vi "Avantes - AVS_PrepareMeasure.vi"(8 "error in (no error)":errorcluster, 11 "Cluster in":T1) -> (0 "error out":errorcluster, 3 "Cluster out":T1)   [LabVIEW 2013, in "Avantes Spectrometer Functions.lvlib"]
uses:
  Avantes Spectrometer Functions.lvlib
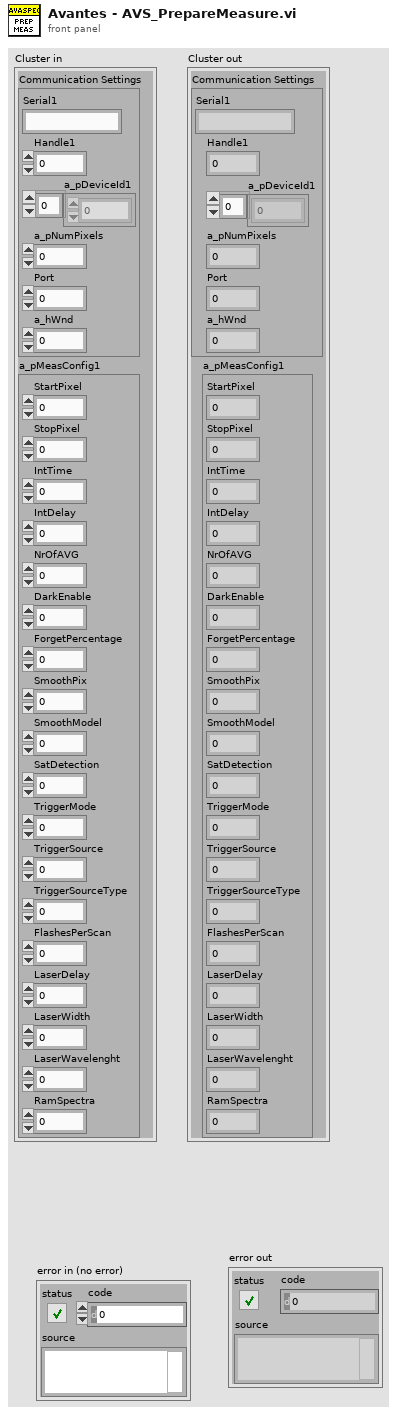
[diagram p1: front panel]
types:
  T1 = cluster{"Communication Settings":cluster{"Serial1":string, "Handle1":i32, "a_pDeviceId1":u8[], "a_pNumPixels":u16, "Port":i32, "a_hWnd":i32}, "a_pMeasConfig1":cluster{"StartPixel":u16, "StopPixel":u16, "IntTime":sgl, "IntDelay":u32, "NrOfAVG":u32, "DarkEnable":u8, "ForgetPercentage":u8, "SmoothPix":u16, "SmoothModel":u8, "SatDetection":u8, "TriggerMode":u8, "TriggerSource":u8, "TriggerSourceType":u8, "FlashesPerScan":u16, "LaserDelay":u32, "LaserWidth":u32, "LaserWavelenght":sgl, "RamSpectra":u16}}
  T2 = cluster{"StartPixel":u16, "StopPixel":u16, "IntTime":sgl, "IntDelay":u32, "NrOfAVG":u32, "DarkEnable":u8, "ForgetPercentage":u8, "SmoothPix":u16, "SmoothModel":u8, "SatDetection":u8, "TriggerMode":u8, "TriggerSource":u8, "TriggerSourceType":u8, "FlashesPerScan":u16, "LaserDelay":u32, "LaserWidth":u32, "LaserWavelenght":sgl, "RamSpectra":u16}
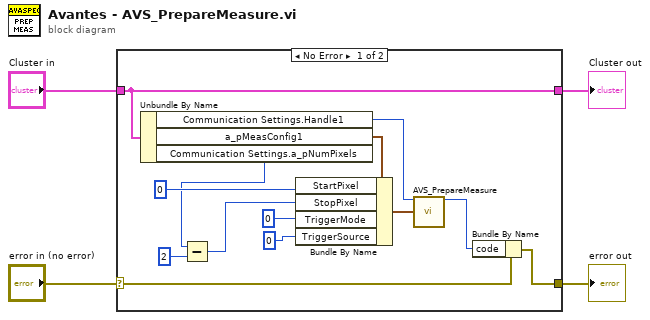
[diagram p0: block diagram]
diagram:
  n1 = case shown="No Error" "error in (no error)" {
    selector: "error in (no error)" -> [w10 w19]
    tunnel: [w11 w18] -> w4
    tunnel: "Cluster in" -> [w11 w18]
    tunnel: [w9 w19] -> w1
    frame No Error {
      n2 = Unbundle By Name(w11) -> ("Communication Settings.Handle1"=w6:i32, "a_pMeasConfig1"=w7:T2, "Communication Settings.a_pNumPixels"=w5:u16)
      n3 = Subtract(x=w5, y=u16 2) -> (x-y=w15:u16)
      n4 = Bundle By Name(cluster=w7, "StartPixel"=0, "StopPixel"=w15, "TriggerMode"=u8 0, "TriggerSource"=u8 0) -> (w17:T2)
      n5 = call "AVS_PrepareMeasure.vi"("a_hDevice"=w6, "a_pMeasConfig"=w17) -> ("Output Value"=w8:i32)  [unwired: 13 in]
      n6 = Bundle By Name(cluster=w10, "code"=w8) -> (w9:errorcluster)
    }
    frame Error {
    }
  }
  "Cluster out" <- w4
  "error out" <- w1
